vi "forward difference.vi"   [LabVIEW 2009, in "common.lvlib"]
uses:
  common.lvlib
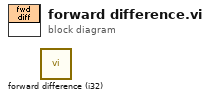
[diagram p0: block diagram]
diagram:
  n1 = call "forward difference (i32).vi"() -> ()  [unwired: 3 in, 1 out]
